vi "Normalize Difference.vi"(9 "data":dbl[][](array[numeric]), 10 "Lower Threshold (% of Min)":dbl=120.0, 11 "Upper Threshold (% of Max)":dbl=80.0) -> (1 "Normalized Difference (Reference - Signal 2)":dbl, 2 "Normalized Difference  (Reference - Signal1)":dbl, 3 "Reference  Normalized Max":dbl)   [LabVIEW 2009]
uses:
  <vilib>/Analysis/6fits.llb/Remove Outliers (Range).vi
  <vilib>/Analysis/NI_AALPro.lvlib
panel:
  out "Normalized Max (Channel Max - Channel Min) 2":dbl
  out "Normalized Max (Channel Max - Channel Min)":dbl
  out "S2/R":dbl
  out "S1/R":dbl
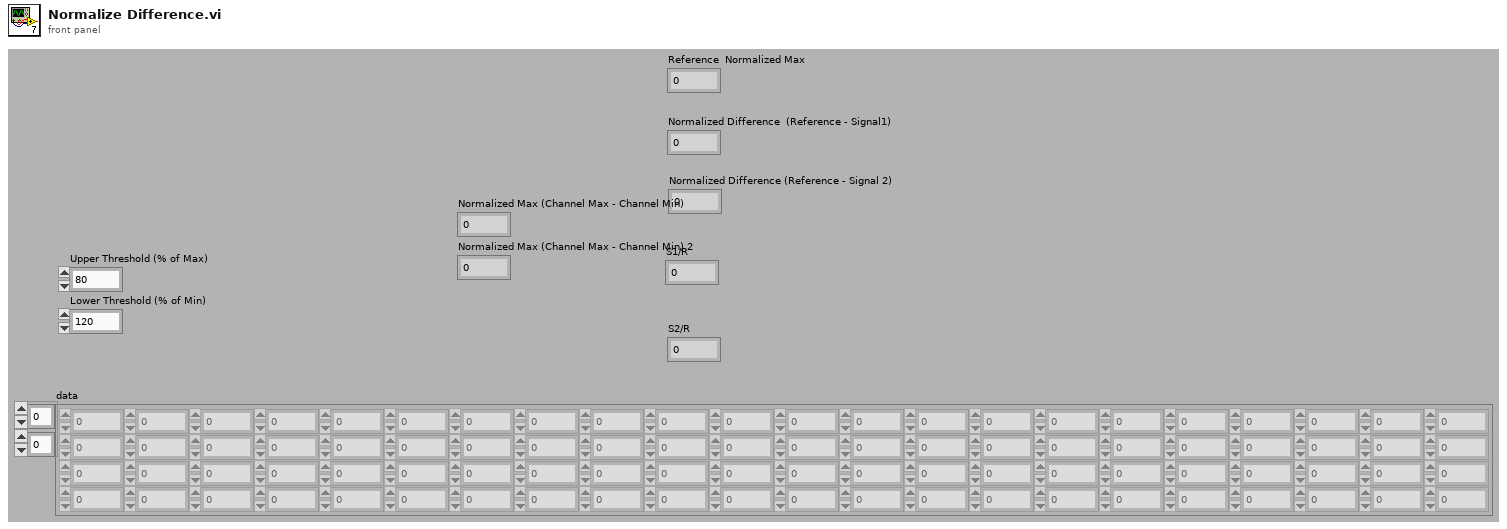
[diagram p1: front panel]
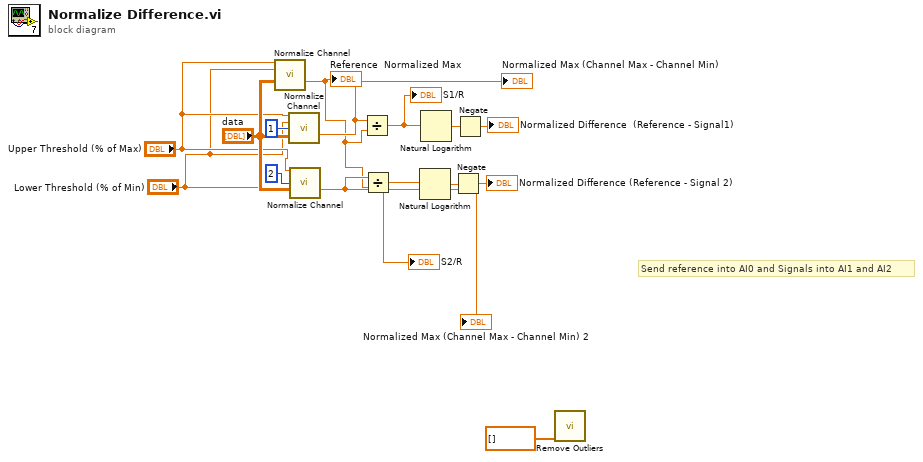
[diagram p0: block diagram]
diagram:
  # "Send reference into AI0 and Signals into AI1 and AI2"
  n1 = call "Normalize Channel.vi"("Upper Threshold (% of Max)"="Upper Threshold (% of Max)", "Lower Threshold (% of Min)"="Lower Threshold (% of Min)", "data"="data") -> ("Normalized Max (Channel Max - Channel Min)"=w4:dbl)  [unwired: 8 in, 4 out]
  "Reference  Normalized Max" <- w4
  n2 = call "Normalize Channel.vi"("Upper Threshold (% of Max)"="Upper Threshold (% of Max)", "Lower Threshold (% of Min)"="Lower Threshold (% of Min)", "index (row)"=1, "data"="data") -> ("Normalized Max (Channel Max - Channel Min)"=w6:dbl)  [unwired: 7 in, 4 out]
  "Normalized Max (Channel Max - Channel Min)" <- w6
  n3 = call "Normalize Channel.vi"("Upper Threshold (% of Max)"="Upper Threshold (% of Max)", "Lower Threshold (% of Min)"="Lower Threshold (% of Min)", "index (row)"=2, "data"="data") -> ("Normalized Max (Channel Max - Channel Min)"=w5:dbl)  [unwired: 7 in, 4 out]
  "Normalized Max (Channel Max - Channel Min) 2" <- w5
  n4 = Divide(x=w6, y=w4) -> (x/y=w2:dbl)
  "S1/R" <- w2
  n5 = Divide(x=w5, y=w4) -> (x/y=w3:dbl)
  "S2/R" <- w3
  n6 = Natural Logarithm(1:w3) -> (0:w15:dbl)
  n7 = Natural Logarithm(1:w2) -> (0:w13:dbl)
  n8 = Negate(x=w15) -> (-x=→"Normalized Difference (Reference - Signal 2)":dbl)
  n9 = Negate(x=w13) -> (-x=→"Normalized Difference  (Reference - Signal1)":dbl)
  n10 = call-poly <vilib>:"Remove Outliers.vi"("Range"=dbl[] []) -> ()  [unwired: 10 in, 5 out]
